vi "Configure Marker Function.vi"(7 "Marker Function":T1, 8 "error in (no error)":errorcluster, 10 "Marker Number (1)":u32=1 min=1, 11 "SA-FSW in":refnum<class "SA-FSW.lvclass">) -> (0 "error out":errorcluster, 3 "SA-FSW out":refnum<class "SA-FSW.lvclass">)   [LabVIEW 2020, in "SA-FSW.lvclass"]
uses:
  SA-FSW.lvclass
  C:/Sandbox/Git_Sandbox/WiSpry Test Framework source code (LV20)/WiSpry Test Framework/Instruments/Instrument.lvclass
  Controls/Marker Functions.ctl
  Instrument.lvclass/Instrument.ctl
  Instrument.lvclass
  Spectrum Analyzer.lvclass
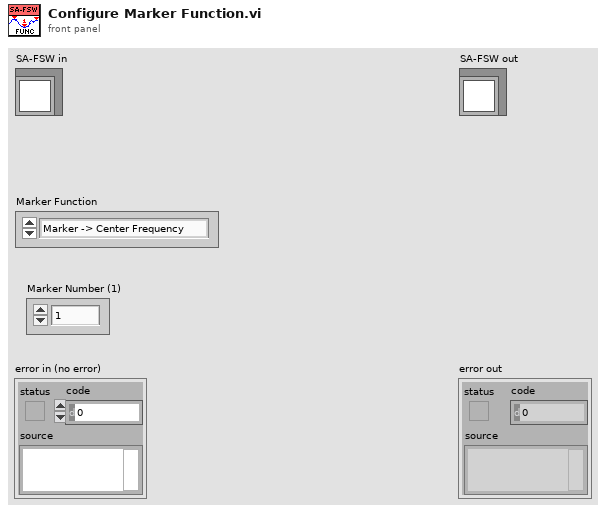
[diagram p1: front panel]
types:
  T1 = typedef "Spectrum Analyzer.lvclass/Marker Functions.ctl" = enum16{"Marker -> Center Frequency", "Marker -> Reference Level"}
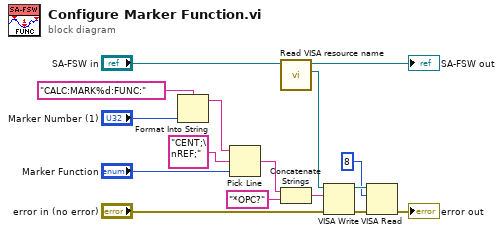
[diagram p0: block diagram]
diagram:
  n1 = Format Into String(format string="CALC:MARK%d:FUNC:", "Marker Number (1)") -> (resulting string=w13:string)  [unwired: 2 in, 1 out]
  n2 = Pick Line(string ("")=w13, multi-line string="CENT;\nREF;", line index="Marker Function") -> (output string=w11:string)
  n3 = call "Read VISA resource name.vi"("Instrument in"="SA-FSW in") -> ("VISA resource name"=w8:refnum<visa-resource-name>, "Instrument out"=→"SA-FSW out":refnum<class "SA-FSW.lvclass">)  [unwired: 9 in]
  n4 = Concatenate Strings(w11, "*OPC?" ("string")) -> (w7:string)
  n5 = VISA Write(VISA resource name=w8, write buffer=w7, error in (no error)="error in (no error)") -> (VISA resource name out=w4:refnum<visa-resource-name>, error out=w5:errorcluster)  [unwired: 1 out]
  n6 = VISA Read(VISA resource name=w4, byte count=u32 8, error in (no error)=w5) -> (error out=→"error out":errorcluster)  [unwired: 3 out]
